vi "Populate Ctrl.vi"(8 "error in (no error)":errorcluster, 11 "PK Field in":refnum<class "PK Field.lvclass">) -> (0 "error out":errorcluster, 3 "PK Field out":refnum<class "PK Field.lvclass">)   [LabVIEW 2020, in "Composed Fields.lvlib" / "PK Field.lvclass"]
uses:
  PK Field.lvclass
  C:/Users/User/Documents/LabVIEW Code/LV-Database-OOP/source/Database OOP/Column Libraries/Column/Composed Column.lvclass
  Ring Ctrl Value Source/Ring Ctrl Value Source.lvclass
  Column/Composed Column.lvclass/Composed Column.ctl
  Composed Columns/Value Source Interface Class/Value Source.lvclass
  Basic Columns/Column Configuration/Basic Column Configuration Class/Column Configuration.lvclass
  Database Libraries/Database Interfaces/Database Interface Class/Database Interface.lvclass
  Column/Composed Column.lvclass
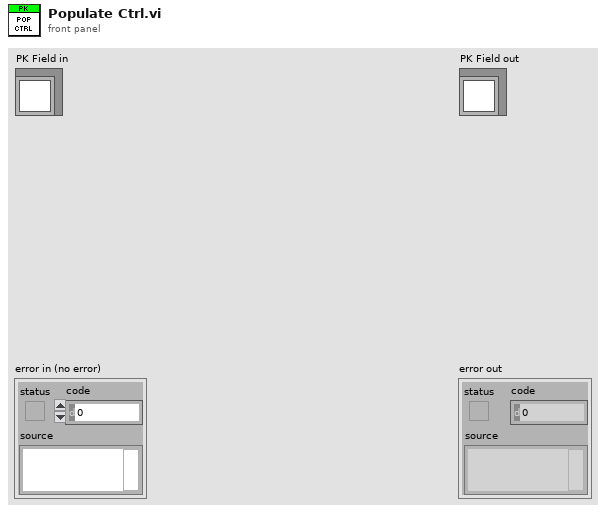
[diagram p1: front panel]
types:
  T1 = typedef "Database Interfaces.lvlib/Primary Key Info.ctl" = cluster{"Primary Key Column":string, "Display Column":string}
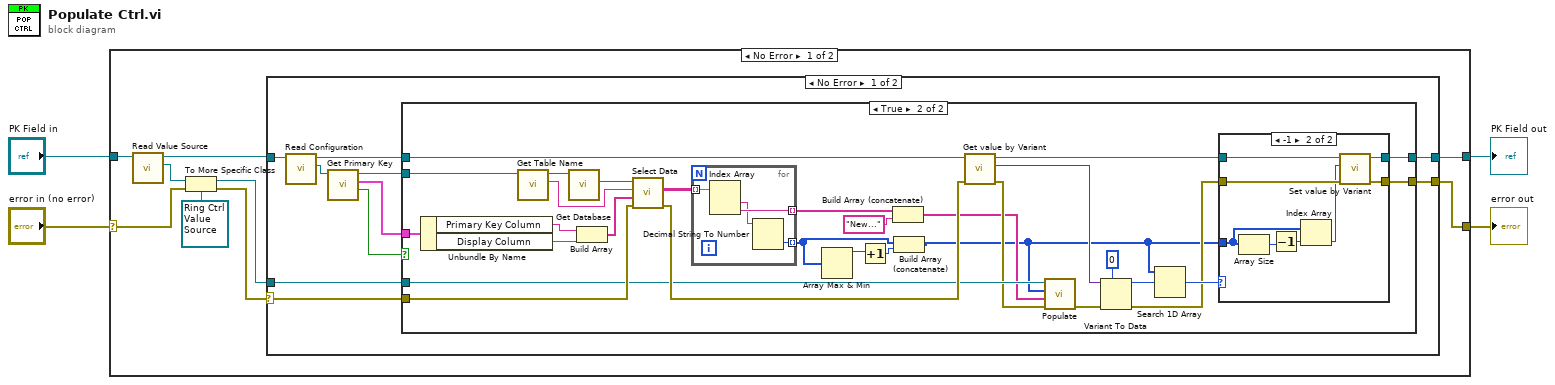
[diagram p0: block diagram]
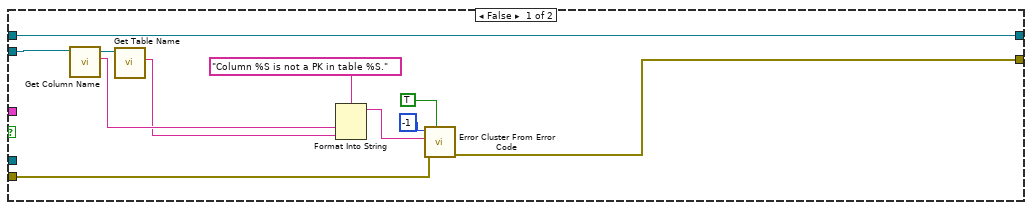
[diagram p2: hidden frame]
diagram:
  n1 = case shown="No Error" "error in (no error)" {
    selector: "error in (no error)" -> [w10 w82]
    tunnel: [w6 w82] -> w1
    tunnel: "PK Field in" -> [w13 w81]
    tunnel: [w5 w81] -> w2
    frame No Error {
      n2 = call "Read Value Source.vi"("Composed Column in"=w13) -> ("Value Source"=w12:refnum<class "Value Source.lvclass">, "Composed Column out"=w9:refnum<class "PK Field.lvclass">)  [unwired: 8 in, 1 out]
      n3 = To More Specific Class(target class=refnum<class "Ring Ctrl Value Source.lvclass"> refnum ("Composed Columns.lvlib:Ring Ctrl Value Source.lvclass"), reference=w12, error in=w10) -> (specific class reference=w7:refnum<class "Ring Ctrl Value Source.lvclass">, error out=w8:errorcluster)
      n4 = case shown="No Error" w8 {
        selector: w8 -> [w23 w79]
        tunnel: [w22 w79] -> w6
        tunnel: w9 -> [w20 w80]
        tunnel: [w21 w80] -> w5
        tunnel: w7 -> [w18 _]
        frame No Error {
          n5 = call "Read Configuration.vi"("Composed Column in"=w20) -> ("Column Interfaces.lvlib:Column Configuration.lvclass"=w17:refnum<class "Column Configuration.lvclass">, "Composed Column out"=w19:refnum<class "PK Field.lvclass">)  [unwired: 8 in, 1 out]
          n6 = call-dynamic "Get Primary Key.vi"("Basic Column Configuration in"=w17) -> ("Is a PK?"=w14:bool, "Primary Key"=w15:T1, "Basic Column Configuration out"=w16:refnum<class "Column Configuration.lvclass">)  [unwired: 7 in, 1 out]
          n7 = case shown="True" w14 {
            tunnel: w16 -> [w25 w44]
            tunnel: w23 -> [w27 w63]
            tunnel: [w26 w58] -> w22
            tunnel: w19 -> [w24 w57]
            tunnel: [w24 w54] -> w21
            tunnel: w15 -> [_ w53]
            tunnel: w18 -> [_ w51]
            frame False {
              n8 = call-dynamic "Get Column Name.vi"("Basic Column Configuration in"=w25) -> ("Column Name"=w32:string, "Basic Column Configuration out"=w33:refnum<class "Column Configuration.lvclass">)  [unwired: 8 in, 1 out]
              n9 = call-dynamic "Get Table Name.vi"("Basic Column Configuration in"=w33) -> ("Table Name"=w31:string)  [unwired: 8 in, 2 out]
              n10 = Format Into String(format string="Column %S is not a PK in table %S.", w32, w31) -> (resulting string=w30:string)  [unwired: 2 in, 1 out]
              n11 = call <vilib>:"Error Cluster From Error Code.vi"("show call chain? (False)"=TRUE, "error in (no error)"=w27, "error message (\"\")"=w30, "error code (0)"=-1) -> ("error out"=w26:errorcluster)  [unwired: 5 in]
            }
            frame True {
              n12 = Unbundle By Name(w53) -> ("Primary Key Column"=w47:string, "Display Column"=w46:string)
              n13 = call-dynamic "Get Table Name.vi"("Basic Column Configuration in"=w44) -> ("Table Name"=w42:string, "Basic Column Configuration out"=w43:refnum<class "Column Configuration.lvclass">)  [unwired: 8 in, 1 out]
              n14 = call-dynamic "Get Database.vi"("Basic Column Configuration in"=w43) -> ("Database"=w64:refnum<class "Database Interface.lvclass">)  [unwired: 8 in, 2 out]
              n15 = Build Array(w47, w46) -> (w45:string[])
              n16 = call-dynamic "Select Data.vi"("error in (no error)"=w63, "Columns"=w45, "Table"=w42, "Database Interface in"=w64) -> ("error out"=w56:errorcluster, "Data"=w62:string[][])  [unwired: 5 in, 1 out]
              n17 = for {
                tunnel: w62 -> [w78] mode=indexing
                tunnel: [w77] -> w38 mode=indexing
                tunnel: [w75] -> w40 mode=indexing
                n18 = Index Array(array=w78) -> (element #1=w76:string, element #2=w77:string)  [unwired: 2 in]
                n19 = Decimal String To Number(string=w76) -> (number=w75:i32)  [unwired: 2 in, 1 out]
              }
              n20 = Array Max & Min(array=w40) -> (max value=w41:i32)  [unwired: 3 out]
              n21 = Increment(x=w41) -> (x+1=w39:i32)
              n22 = Build Array (concatenate)(w38, "New...") -> (w36:string[])
              n23 = Build Array (concatenate)(w40, w39) -> (w35:i32[])
              n24 = call-dynamic "Get value by Variant.vi"("error in (no error)"=w56, "Column in"=w57) -> ("error out"=w50:errorcluster, "Variant"=w55:variant, "Column out"=w52:refnum<class "PK Field.lvclass">)  [unwired: 6 in, 1 out]
              n25 = call-dynamic "Populate.vi"("error in (no error)"=w50, "Display Text Array"=w36, "Values Array"=w35, "Ring Ctrl Value Source in"=w51) -> ("error out"=w49:errorcluster)  [unwired: 6 in, 1 out]
              n26 = Variant To Data(error in=w49, type=0, Variant=w55) -> (data=w60:i32, error out=w48:errorcluster)
              n27 = Search 1D Array(1D array=w35, element=w60) -> (index of element=w59:i32)  [unwired: 1 in]
              n28 = case shown="-1" w59 {
                tunnel: w35 -> [_ w70]
                tunnel: w48 -> [w66 w72]
                tunnel: [w66 w71] -> w58
                tunnel: w52 -> [w65 w74]
                tunnel: [w65 w73] -> w54
                frame 0, Default {
                }
                frame -1 {
                  n29 = Array Size(array=w70) -> (size(s)=w68:i32)
                  n30 = Decrement(x=w68) -> (x-1=w67:i32)
                  n31 = Index Array(array=w70, index=w67) -> (element=w69:i32)
                  n32 = call-dynamic "Set value by Variant.vi"("error in (no error)"=w72, "Variant"=w69, "Column in"=w74) -> ("error out"=w71:errorcluster, "Column out"=w73:refnum<class "PK Field.lvclass">)  [unwired: 7 in]
                }
              }
            }
          }
        }
        frame Error {
        }
      }
    }
    frame Error {
    }
  }
  "error out" <- w1
  "PK Field out" <- w2
